vi "scale data trial.vi"() -> ()   [LabVIEW 2018]
uses:
  RT/Type Defs/Data processing loop data.ctl
  RT/Type Defs/FPGA reference.ctl
  RT/Type Defs/channelCalibration.ctl
  RT/Type Defs/channelScalingTypes.ctl
  RT/Type Defs/scalingMethods.ctl
panel:
  in  "input cluster":T1={"Parameters"={"FPGA Ref"=refnum, "data stream"={"data writer name"="error writer", "NS write buffer size"=16, "NS Buffer length"=0}, "FIFO Depth"=0, "Channel controls"={"FIFIO channel count"=0, "active indices"=[], "active channels"=0, "channelScaling"=[], "scanivalveCount"=0}, "safetyChannels"={"oilP"=0, "airP"=0, "water"=0, "temperatures"=[]}}, "Variables"={"Intermediary buffer"=[], "buffer position"=0, "write loop counter"=0, "NS write trigger"=0, "NS Connection status"=FALSE, "waiting for NS"=FALSE, "labAmbient"={"pressure"=0.0, "temperature"=0.0}, "scanivalvePorts"=[], "scanivalvePressures"=[], "data stream"=""}}
  out "time":dbl
  out "Data received":sgl[][](array[numeric])
  out "data length":i32
  out "Active channels":sgl[][](array[numeric])
  in  "raw data":sgl[](array[numeric])=array[88682 elements]
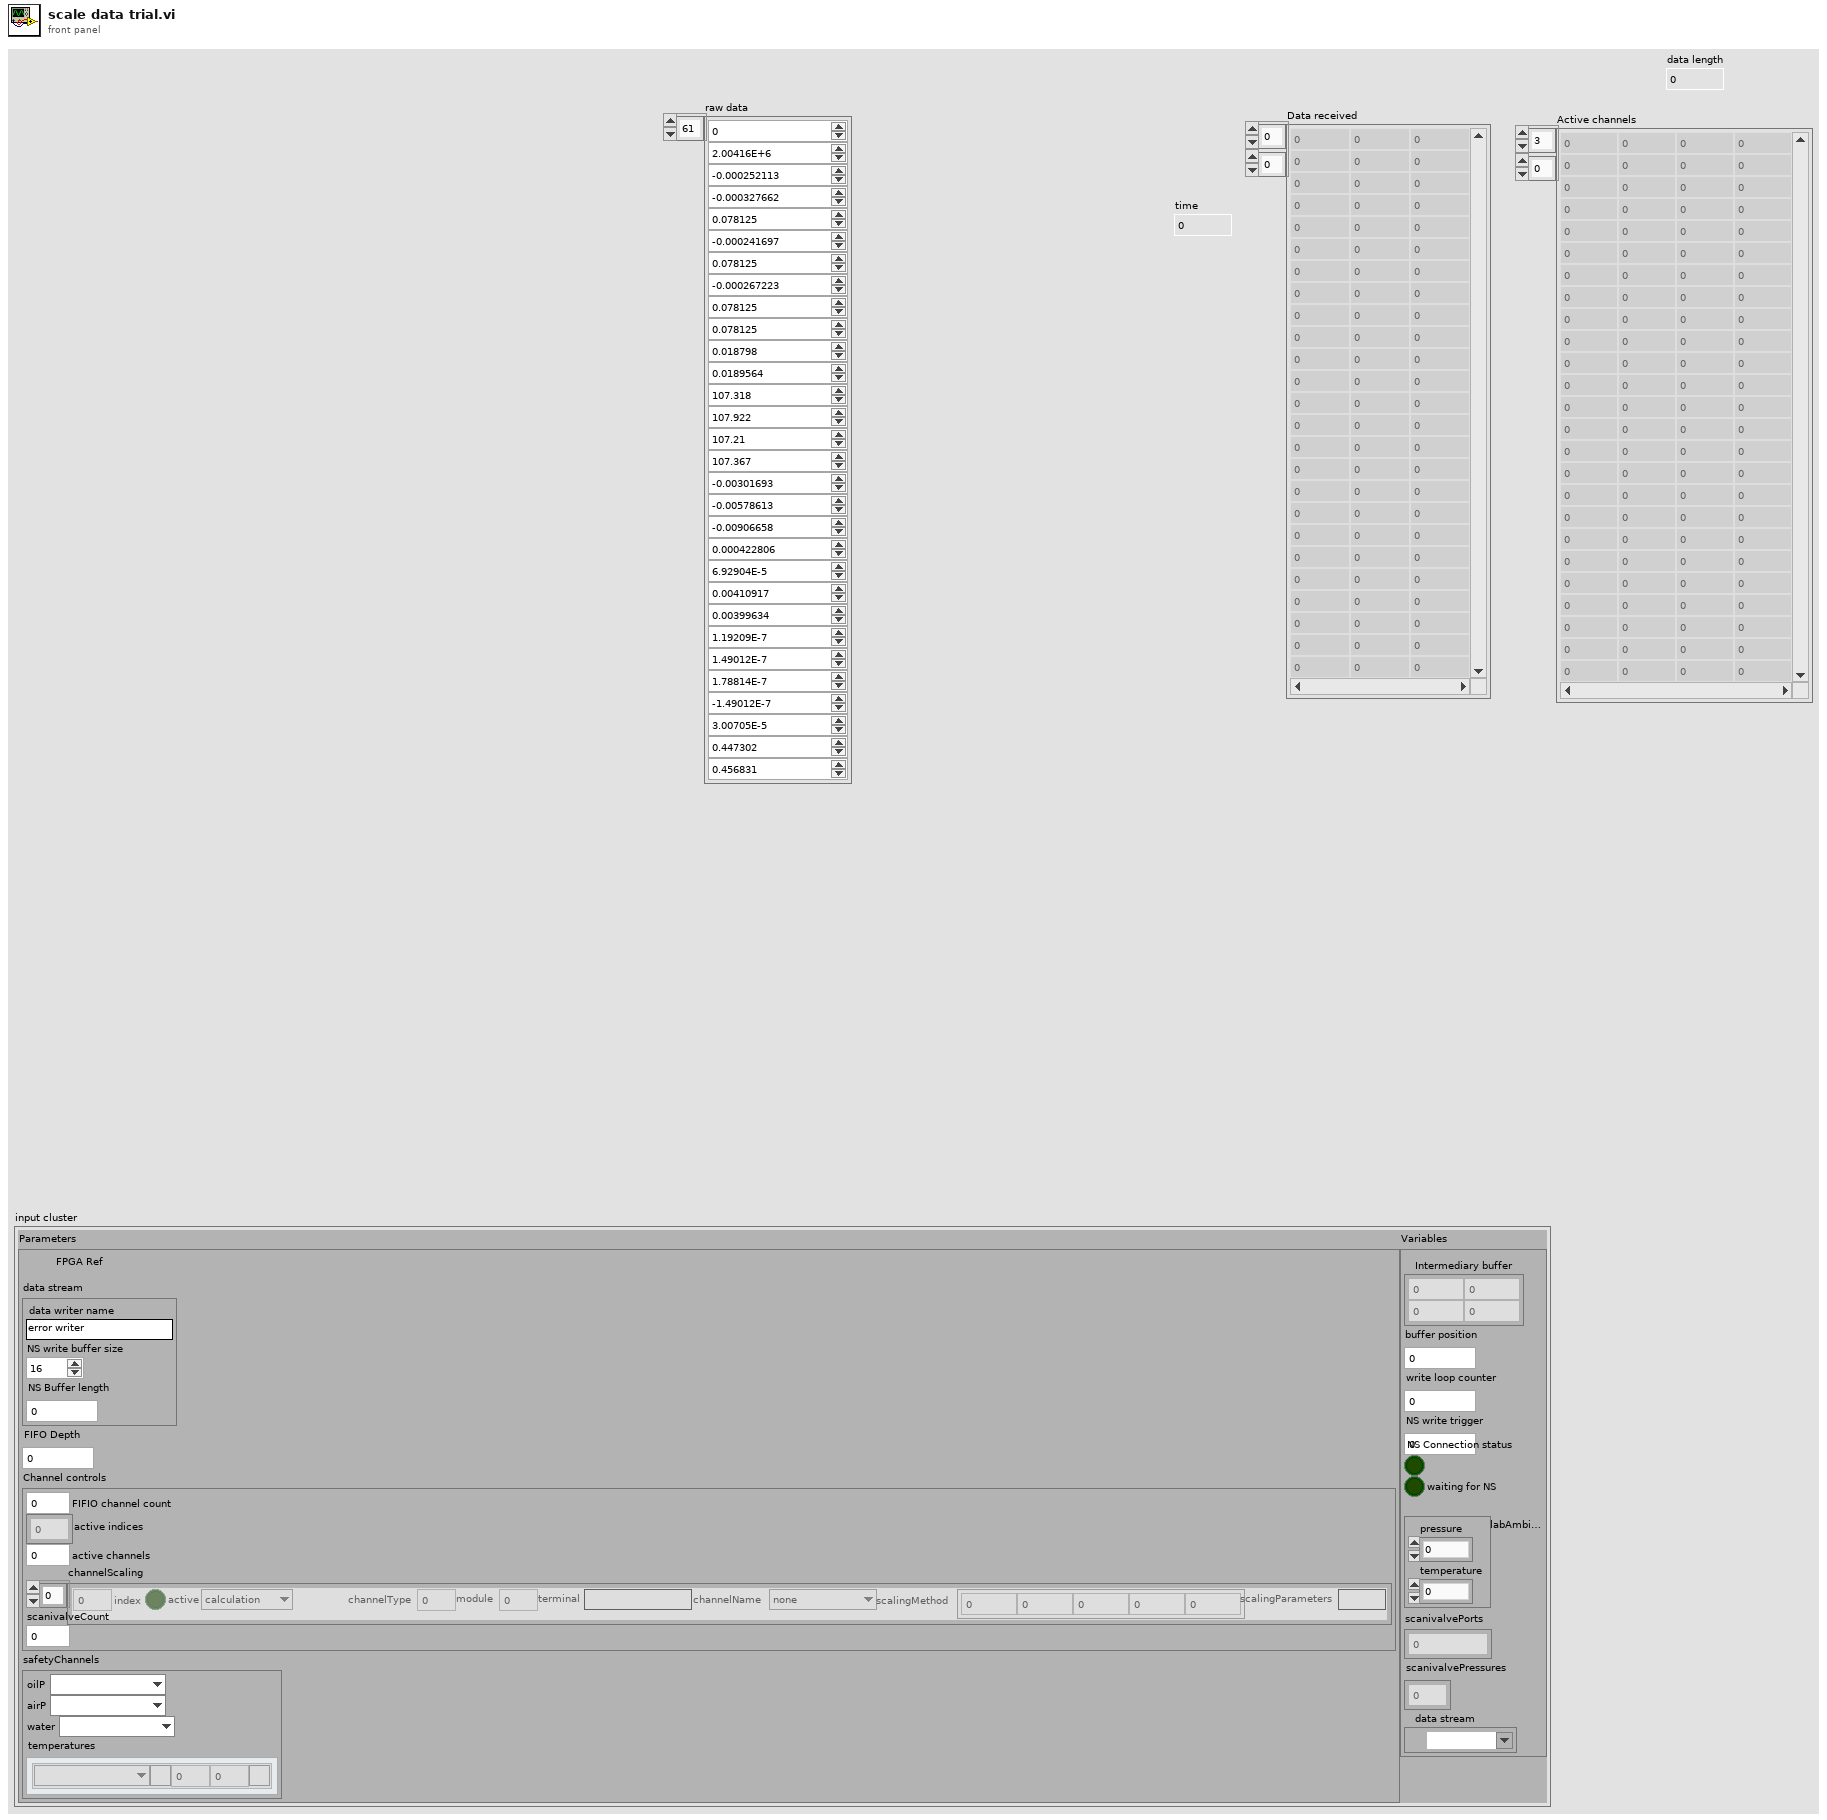
[diagram p1: front panel]
types:
  T1 = typedef "Data processing loop data.ctl" = cluster{"Parameters":cluster{"FPGA Ref":T2, "data stream":cluster{"data writer name":string, "NS write buffer size":i32, "NS Buffer length":u32}, "FIFO Depth":u32, "Channel controls":cluster{"FIFIO channel count":i32, "active indices":i16[], "active channels":i32, "channelScaling":T3[], "scanivalveCount":i32}, "safetyChannels":cluster{"oilP":u16, "airP":u16, "water":u16, "temperatures":cluster{"Oil pressure: 4":u16, "Enabled":bool, "warning temp":dbl, "limit temp":dbl, "Invert":bool}[]}}, "Variables":cluster{"Intermediary buffer":dbl[][], "buffer position":u32, "write loop counter":u16, "NS write trigger":u32, "NS Connection status":bool, "waiting for NS":bool, "labAmbient":cluster{"pressure":dbl, "temperature":dbl}, "scanivalvePorts":u16[], "scanivalvePressures":dbl[], "data stream":refnum<k21>}}
  T2 = typedef "FPGA reference.ctl" = refnum<k20>
  T3 = typedef "channelCalibration.ctl" = cluster{"index":u16, "active":bool, "channelType":T4, "module":u16, "terminal":u16, "channelName":string, "scalingMethod":T5, "scalingParameters":dbl[], "scaledUnits":string}
  T4 = typedef "channelScalingTypes.ctl" = enum16{"calculation", "measurement", "scanivalve", "output", "digital"}
  T5 = typedef "scalingMethods.ctl" = enum16{"none", "linear", "thermocouple", "polynomial", "encoder", "RTD"}
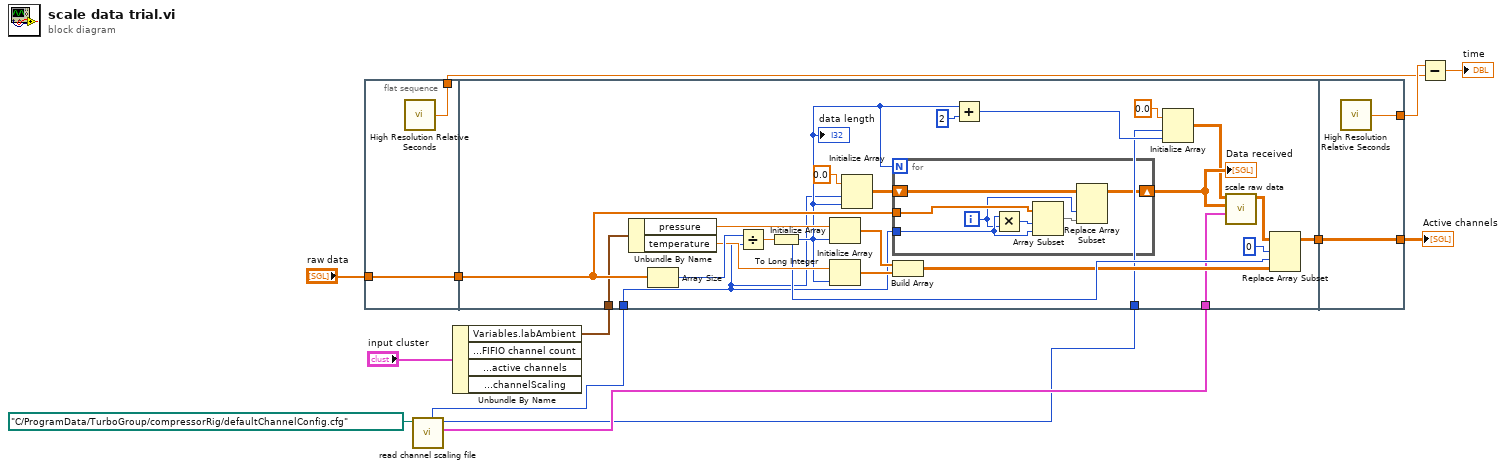
[diagram p0: block diagram]
diagram:
  n1 = flat-sequence {
    tunnel: "raw data" -> [w15]
    tunnel: [w15] -> w13
    tunnel: [w14] -> w8
    tunnel: w13 -> [w35]
    tunnel: [w25] -> w12
    tunnel: w1 -> [w19]
    tunnel: w2 -> [w18]
    tunnel: w5 -> [w17]
    tunnel: w4 -> [w16]
    tunnel: [w47] -> w10
    tunnel: w12 -> [w47]
    tunnel: [w46] -> w9
    frame #0 {
      n2 = call <vilib>:"High Resolution Relative Seconds.vi"() -> ("relative seconds"=w14:dbl)
    }
    frame #1 {
      n3 = Unbundle By Name(w17) -> ("pressure"=w29:dbl, "temperature"=w28:dbl)
      n4 = Array Size(array=w35) -> (size(s)=w38:i32)
      n5 = Divide(x=w38, y=w19) -> (x/y=w37:dbl)
      n6 = To Long Integer(number=w37) -> (32bit integer=w24:i32)
      "data length" <- w24
      n7 = Initialize Array(w29, w24) -> (w23:dbl[])
      n8 = Initialize Array(w28, w24) -> (w22:dbl[])
      n9 = Initialize Array(sgl 0.0 ("raw data"), w19, w24) -> (w34:sgl[][])
      n10 = for {
        N: w24 -> [_]
        tunnel: w35 -> [w45]
        shift-right: [w40] -> w33
        shift-left: w34 -> [w42]
        tunnel: w19 -> [w43]
        i -> [w39]
        n11 = Multiply(x=w43, y=w39) -> (x*y=w44:i32)
        n12 = Array Subset(array=w45, index=w44, length=w43) -> (w41:sgl[])
        n13 = Replace Array Subset(array=w42, new element=w41, index (col)=w39) -> (w40:sgl[][])  [unwired: 1 in]
      }
      "Data received" <- w33
      n14 = Build Array(w23, w22) -> (w21:dbl[][])
      n15 = Add(x=w24, y=2) -> (x+y=w27:i32)
      n16 = Initialize Array(sgl 0.0 ("raw data"), w18, w27) -> (w31:sgl[][])
      n17 = call "scale raw data.vi"("channelScaling"=w16, "raw data"=w33, "scaled data"=w31) -> ("scaled data"=w30:dbl[][])  [unwired: 8 in]
      n18 = Replace Array Subset(array=w30, new element=w21, index (row)=0 ("disabled index (row)"), index (col)=w24) -> (w25:dbl[][])
    }
    frame #2 {
      n19 = call <vilib>:"High Resolution Relative Seconds.vi"() -> ("relative seconds"=w46:dbl)
    }
  }
  n20 = call "read channel scaling file.vi"("file path"=path "C:/ProgramData/TurboGroup/compressorRig/defaultChannelConfig.cfg") -> ("channelConfig"=w4:T3[], "activeChannelCount"=w2:u16, "FIFO channels"=w1:u16)  [unwired: 6 in, 2 out]
  n21 = Unbundle By Name("input cluster") -> ("Variables.labAmbient"=w5:cluster{"pressure":dbl, "temperature":dbl})  [unwired: 3 out]
  n22 = Subtract(x=w9, y=w8) -> (x-y=→"time":dbl)
  "Active channels" <- w10
